vi "VibratomeGUI.vi"() -> ()   [LabVIEW 2014]
uses:
  Hardware/Table Stage/Controls/Translation Stage Cluster.ctl
  General/Controls/Translation Stage Types.ctl
  General/Controls/Translation Stage Quick Status.ctl
  General/Controls/Translation Stage Quick Controls.ctl
  General/Controls/Queue Manager Actions.ctl
  General/Controls/MessagePacket.ctl
  General/Controls/QueueNames.ctl
  <vilib>/Utility/miscctls.llb/LVPointTypeDef.ctl
  Hardware/Table Stage/Controls/Motion Translation Module Control.ctl
  General/Controls/Set Get Controls.ctl
panel:
  in  "Z STEP MOTION":enum16{"Fine", "Course", "Extra Course"}(ring)
  in  "Stop Button":bool
  in  "Slice":bool
  in  "Vibratome Controls":T1
  out "Message":string
  in  "Z Ctrl":T2
  out "Z Status":T3
  in  "Y Ctrl":T2
  out "Y Status":T3
  in  "X Ctrl":T2
  out "X Status":T3
  in  "XY STEP MOTION":enum16{"Fine", "Course", "Extra Course"}(ring)
  out "Cluster":cluster{"X":T4, "Y":T4, "Z":T4}
  in  "Exit":bool
  out "Processor Error Out":errorcluster
  out "GUI Error Out":errorcluster
  # "Vibratome Controls"
  # "Z Axis"
  # "Y Axis"
  # "X Axis"
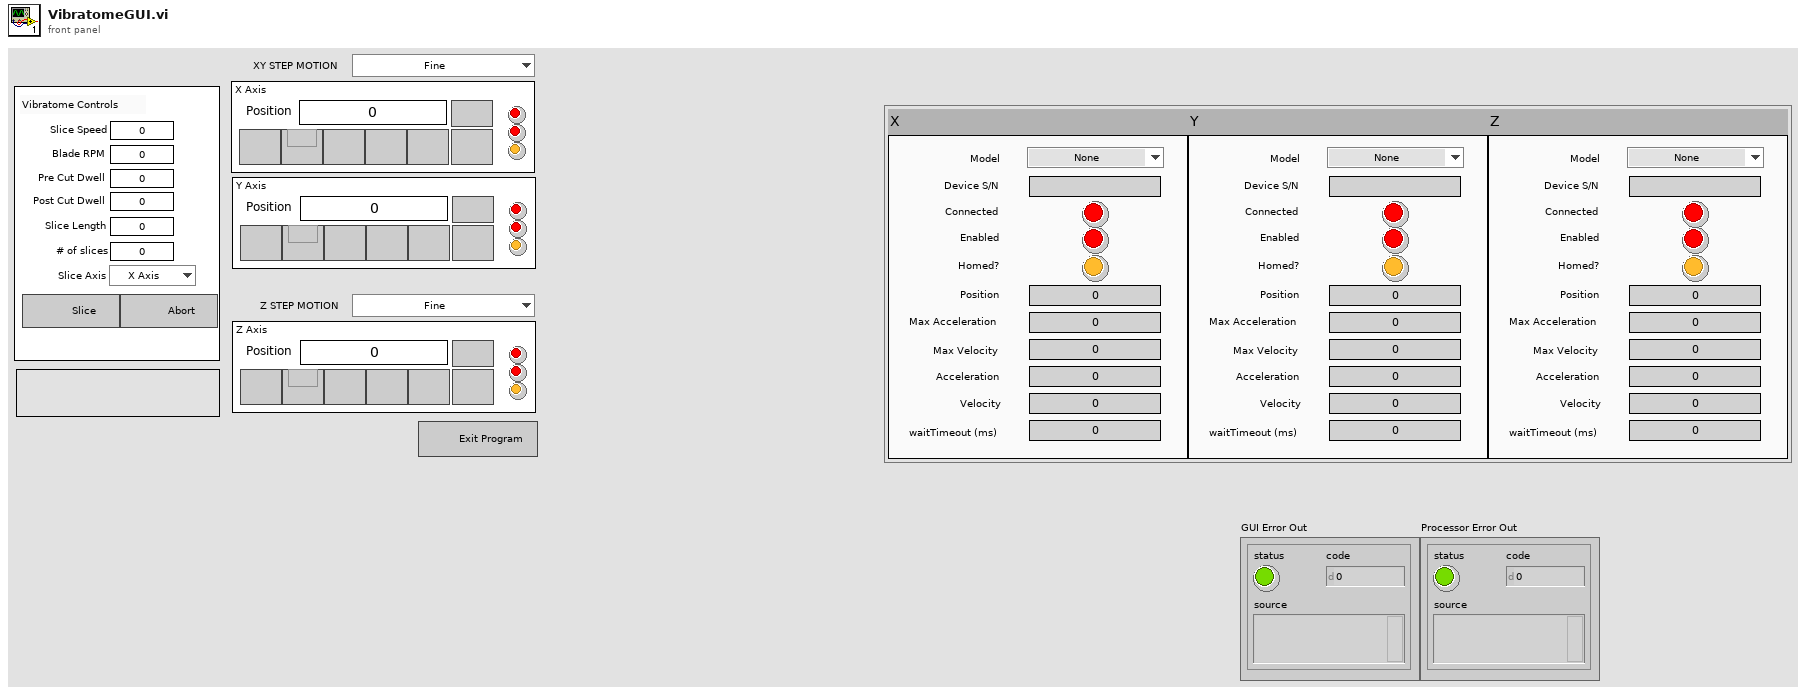
[diagram p1: front panel]
types:
  T1 = cluster{"Pre Cut Dwell":dbl, "Blade RPM":u16, "Slice Speed":dbl, "Post Cut Dwell":dbl, "Slice Length":dbl, "# of slices":dbl, "Slice Axis":enum16{"X Axis", "Y Axis", "Z Axis"}}
  T2 = typedef "Translation Stage Quick Controls.ctl" = cluster{"Position":dbl, "Next Button":bool, "Last Button":bool, "Previous Button":bool, "First Button":bool, "Home Button":bool, "Go":bool, "Settings Button":bool}
  T3 = typedef "Translation Stage Quick Status.ctl" = cluster{"Is.Enabled?":bool, "Is.Connected?":bool, "Is.Homed?":bool}
  T4 = typedef "Translation Stage Cluster.ctl" = cluster{"Position":dbl, "Is.Enabled?":bool, "Is.Connected?":bool, "Device SN":string, "AccelerationMaximum":dbl, "VelocityMaximum":dbl, "Acceleration":dbl, "Velocity":dbl, "waitTimeout (ms)":i32, "Model":T5, "Is.Homed?":bool}
  T5 = typedef "Translation Stage Types.ctl" = enum16{"None", "Thorlabs LTS", "Thorlabs MLJ"}
  T6 = typedef "MessagePacket.ctl" = cluster{"Message":string, "Parameter":variant}
  T7 = typedef "Queue Manager Actions.ctl" = enum16{"Init", "Enqueue", "Enqueue All", "Preview Queue", "Dequeue", "Get Status", "Flush Queue", "Flush All Queues", "Release All Queues", "Release Queue", "Enqueue at Opposite End"}
  T8 = typedef "QueueNames.ctl" = enum16{"Main GUI", "Main Scan Processor", "Main Display", "Main Table Stage GUI", "Main Table Stage Proc.", "Scan Engine", "Vibratome GUI", "Vibratome Processor", "Slice Engine"}
  T9 = typedef "LVPointTypeDef.ctl" = cluster{"Horizontal":i16, "Vertical":i16}
  T10 = enum16{"Set Configuration", "Get Configuration", "Enable Motor", "Disable Motor", "Get Status", "Open Session", "Close Session", "Set Limits", "Get Limits"}
  T11 = typedef "Set Get Controls.ctl" = enum16{"Set", "Get"}
  T12 = typedef "Motion Translation Module Control.ctl" = enum16{"Init", "Home", "Status", "Velocity/Accel", "Position", "Jog", "Stop", "Uninit", "Enable", "Disable"}
  T13 = cluster{"X Stage":T4, "Y Stage":T4, "Z Stage":T4}
  T14 = typedef "System Parameters.ctl" = cluster{"OCT":cluster{"Focal Length":dbl[unit]}, "Vibratome":cluster{"Z Bottom [mm]":dbl, "Pre Cut Dwell [s]":dbl, "Blade Frequency [RPM]":u16, "Slice Speed [mm/s]":dbl, "Post Cut Dwell [s]":dbl, "Ramp Time [s]":dbl, "Start X [mm]":dbl, "Start Y [mm]":dbl, "Slice Length [mm]":dbl, "Slice Axis":enum16{"X Axis", "Y Axis", "Z Axis"}, "Controller VISA Ref":refnum<visa-resource-name>}, "Table Stages":cluster{"X Stage":T4, "Y Stage":T4, "Z Stage":T4}}
  T15 = cluster{"Z Bottom [mm]":dbl, "Pre Cut Dwell [s]":dbl, "Blade Frequency [RPM]":u16, "Slice Speed [mm/s]":dbl, "Post Cut Dwell [s]":dbl, "Ramp Time [s]":dbl, "Start X [mm]":dbl, "Start Y [mm]":dbl, "Slice Length [mm]":dbl, "Slice Axis":enum16{"X Axis", "Y Axis", "Z Axis"}, "Controller VISA Ref":refnum<visa-resource-name>}
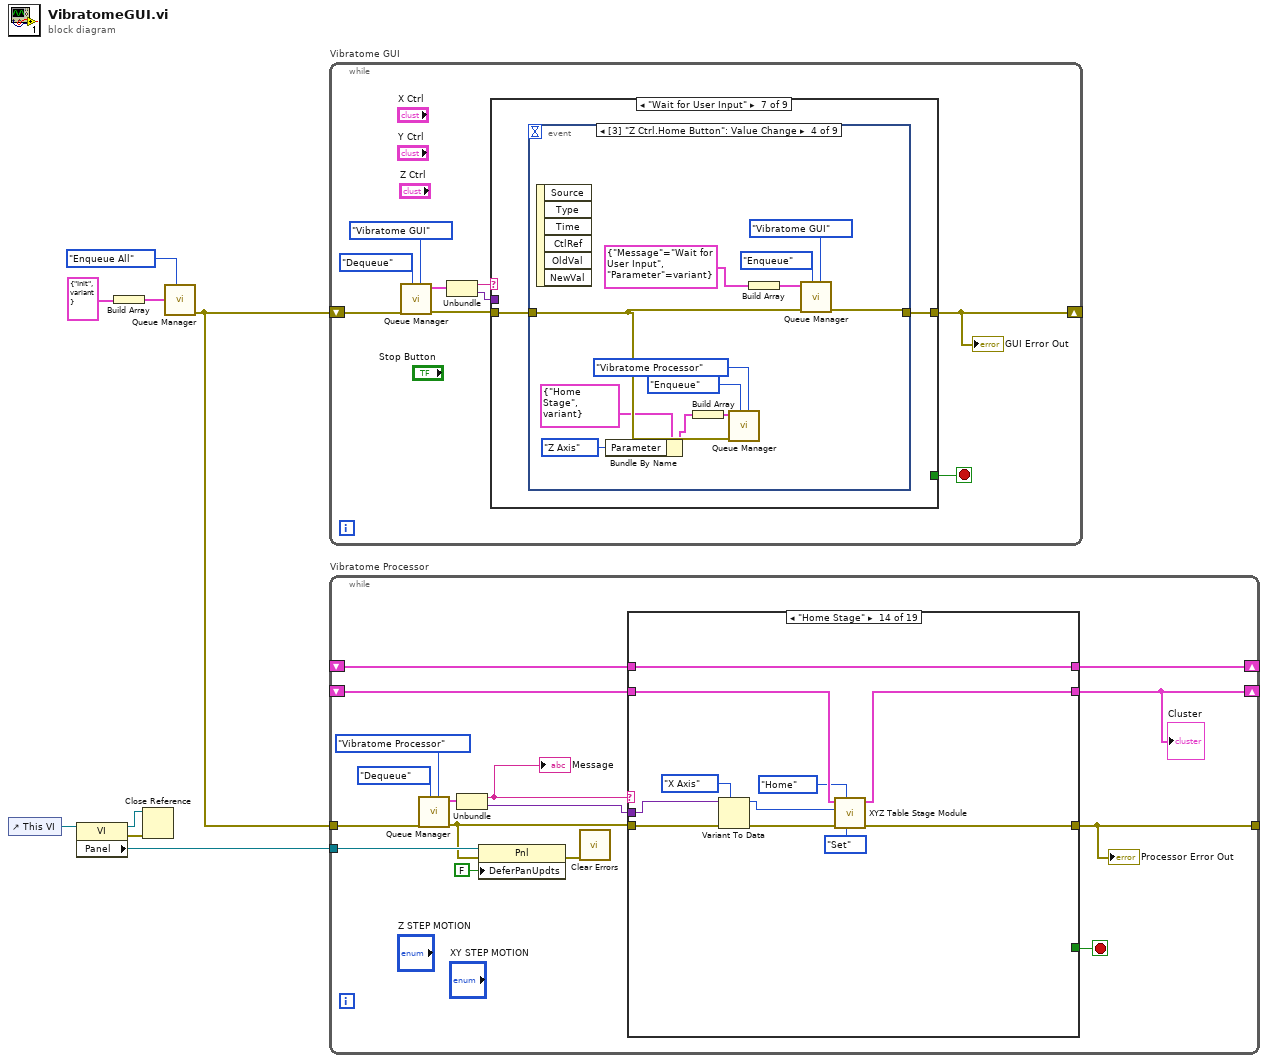
[diagram p0: block diagram]
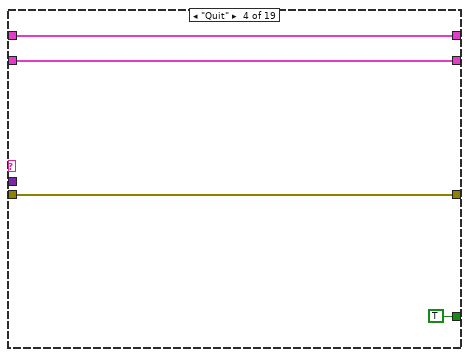
[diagram p5: hidden frame]
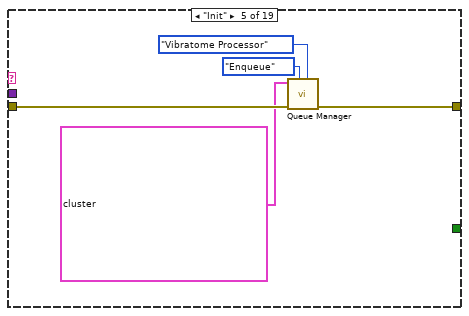
[diagram p6: hidden frame]
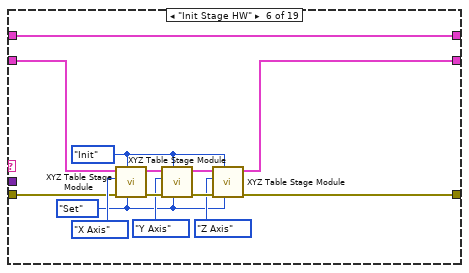
[diagram p7: hidden frame]
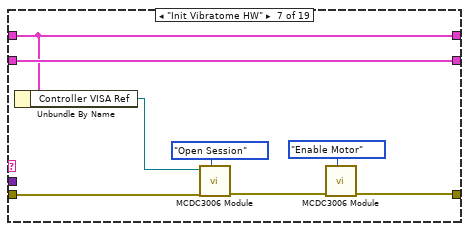
[diagram p8: hidden frame]
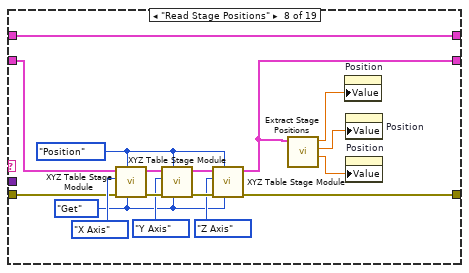
[diagram p9: hidden frame]
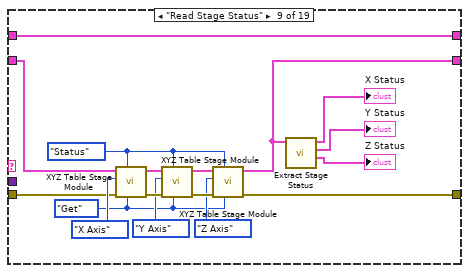
[diagram p10: hidden frame]
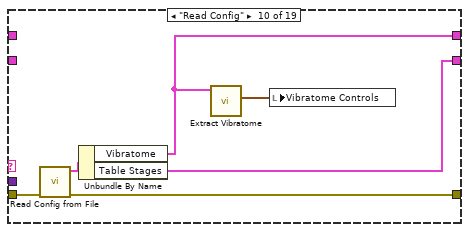
[diagram p11: hidden frame]
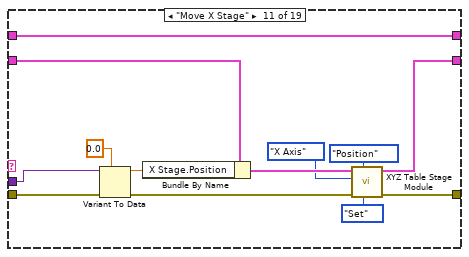
[diagram p12: hidden frame]
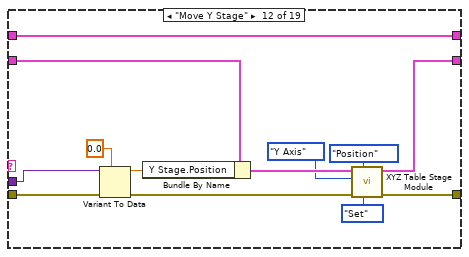
[diagram p13: hidden frame]
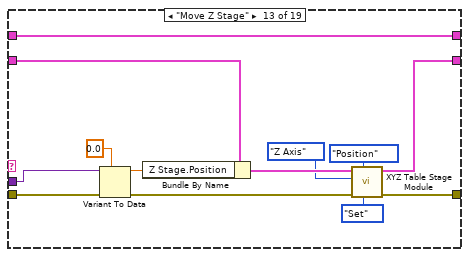
[diagram p14: hidden frame]
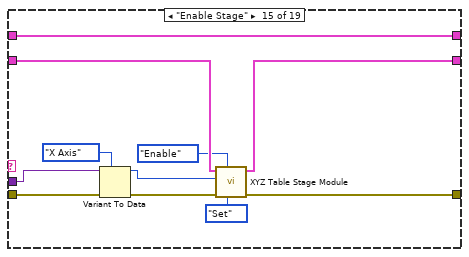
[diagram p15: hidden frame]
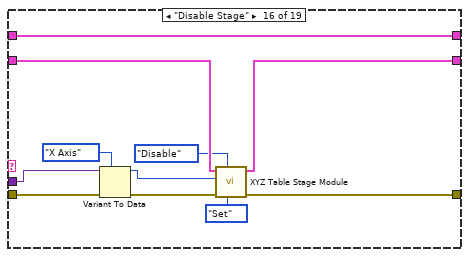
[diagram p16: hidden frame]
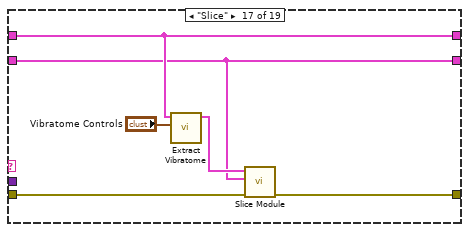
[diagram p17: hidden frame]
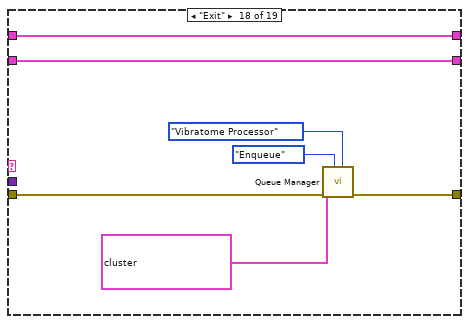
[diagram p18: hidden frame]
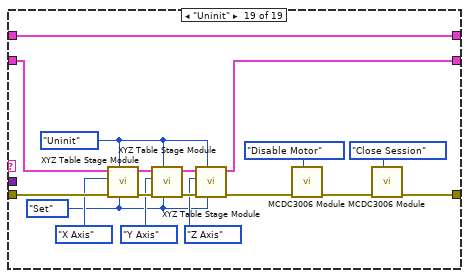
[diagram p19: hidden frame]
diagram:
  n1 = control-ref of="This VI"() -> (w4:refnum<vi>)
  n2 = property class="VI"(reference=w4) -> (reference out=w2:refnum<vi>, error out=w3:errorcluster, "Panel"=w1:refnum<vi>)  [unwired: 1 in]
  n3 = Build Array(T6 {"Message"="Init", "Parameter"=variant} ("Message Packet [In]")) -> (w6:T6[])
  n4 = Close Reference(reference=w2, error in (no error)=w3) -> ()  [unwired: 1 out]
  n5 = call "Queue Manager.vi"("Action"=Queue_Manager_Actions."Enqueue All", "Message Packet Array"=w6) -> ("Error Out"=w5:errorcluster)  [unwired: 7 in, 2 out]
  n6 = while "Vibratome GUI" {
    shift-right: [w17] -> _
    shift-left: w5 -> [w15]
    stop <- w10 stop-if-true
    n7 = call "Queue Manager.vi"("Queue Name"=QueueNames."Vibratome GUI", "Action"=Queue_Manager_Actions."Dequeue", "Error In"=w15) -> ("Error Out"=w14:errorcluster, "Message Packet [Out]"=w13:T6)  [unwired: 6 in, 1 out]
    n8 = Unbundle(w13) -> ("Message"=w12:string, "Parameter"=w11:variant)
    n9 = case shown="\"Wait for User Input\"" w12 {
      tunnel: w14 -> [w18 w19 w24 w25 w26 w27 w29 w126 w139]
      tunnel: [w18 w20 w24 w25 w26 w27 w28 w127 w139] -> w17
      tunnel: w11 -> [_ _ _ _ _ _ _ _ _]
      tunnel: [_ _ _ _ _ _ _ _ TRUE] -> w10
      frame "Unknown", Default {
      }
      frame "Init" {
        n10 = call "Queue Manager.vi"("Queue Name"=QueueNames."Vibratome GUI", "Action"=Queue_Manager_Actions."Enqueue", "Error In"=w19, "Message Packet Array"=T6[] [{"Message"="Init Variables", "Parameter"=variant}, {"Message"="Set Front Panel", "Parameter"=variant}, {"Message"="Load User Settings", "Parameter"=variant}, {"Message"="Configure Hardware", "Parameter"=variant}, {"Message"="Wait for Complete", "Parameter"=variant}, {"Message"="Wait for User Input", "Parameter"=variant}]) -> ("Error Out"=w20:errorcluster)  [unwired: 5 in, 2 out]
      }
      frame "Init Variables" {
      }
      frame "Load User Settings" {
      }
      frame "Configure Hardware" {
      }
      frame "Wait for Complete" {
      }
      frame "Wait for User Input" {
        n11 = event shown="[3] \"Z Ctrl.Home Button\": Value Change" {
          selector: _ -> [_ _ _ _ _ _ _ _ _]
          dyn-events: _ -> [_ _ _ _ _ _ _ _ _]
          timeout: _ -> [_ _ _ _ _ _ _ _ _]
          tunnel: w29 -> [w30 w38 w50 w62 w70 w73 w95 w110 w125]
          tunnel: [w30 w37 w49 w61 w69 w78 w82 w97 w112] -> w28
          event Timeout {
            n12 = event-data() -> ()  [unwired: 1 in, 3 out]
          }
          event Value Change {
            n13 = event-data() -> ()  [unwired: 1 in, 6 out]
            n14 = Bundle By Name(cluster=T6 {"Message"="Home Stage", "Parameter"=variant} ("Message Packet [In]"), "Parameter"=enum16{"X Axis", "Y Axis", "Z Axis"}."X Axis" ("Axis")) -> (w32:T6)
            n15 = Build Array(w32) -> (w33:T6[])
            n16 = call "Queue Manager.vi"("Queue Name"=QueueNames."Vibratome Processor", "Action"=Queue_Manager_Actions."Enqueue", "Error In"=w38, "Message Packet Array"=w33) -> ()  [unwired: 5 in, 3 out]
            n17 = Build Array(T6 {"Message"="Wait for User Input", "Parameter"=variant} ("Message Packet [In]")) -> (w35:T6[])
            n18 = call "Queue Manager.vi"("Queue Name"=QueueNames."Vibratome GUI", "Action"=Queue_Manager_Actions."Enqueue", "Error In"=w38, "Message Packet Array"=w35) -> ("Error Out"=w37:errorcluster)  [unwired: 5 in, 2 out]
          }
          event Value Change {
            n19 = event-data() -> ()  [unwired: 1 in, 6 out]
            n20 = Bundle By Name(cluster=T6 {"Message"="Home Stage", "Parameter"=variant} ("Message Packet [In]"), "Parameter"=enum16{"X Axis", "Y Axis", "Z Axis"}."Y Axis" ("Axis")) -> (w44:T6)
            n21 = Build Array(w44) -> (w45:T6[])
            n22 = call "Queue Manager.vi"("Queue Name"=QueueNames."Vibratome Processor", "Action"=Queue_Manager_Actions."Enqueue", "Error In"=w50, "Message Packet Array"=w45) -> ()  [unwired: 5 in, 3 out]
            n23 = Build Array(T6 {"Message"="Wait for User Input", "Parameter"=variant} ("Message Packet [In]")) -> (w47:T6[])
            n24 = call "Queue Manager.vi"("Queue Name"=QueueNames."Vibratome GUI", "Action"=Queue_Manager_Actions."Enqueue", "Error In"=w50, "Message Packet Array"=w47) -> ("Error Out"=w49:errorcluster)  [unwired: 5 in, 2 out]
          }
          event Value Change {
            n25 = event-data() -> ()  [unwired: 1 in, 6 out]
            n26 = Bundle By Name(cluster=T6 {"Message"="Home Stage", "Parameter"=variant} ("Message Packet [In]"), "Parameter"=enum16{"X Axis", "Y Axis", "Z Axis"}."Z Axis" ("Axis")) -> (w56:T6)
            n27 = Build Array(w56) -> (w57:T6[])
            n28 = call "Queue Manager.vi"("Queue Name"=QueueNames."Vibratome Processor", "Action"=Queue_Manager_Actions."Enqueue", "Error In"=w62, "Message Packet Array"=w57) -> ()  [unwired: 5 in, 3 out]
            n29 = Build Array(T6 {"Message"="Wait for User Input", "Parameter"=variant} ("Message Packet [In]")) -> (w59:T6[])
            n30 = call "Queue Manager.vi"("Queue Name"=QueueNames."Vibratome GUI", "Action"=Queue_Manager_Actions."Enqueue", "Error In"=w62, "Message Packet Array"=w59) -> ("Error Out"=w61:errorcluster)  [unwired: 5 in, 2 out]
          }
          event Panel Close; Application Instance Close; "Exit": Value Change {
            n31 = event-data() -> ()  [unwired: 1 in, 3 out]
            n32 = Build Array(T6 {"Message"="Exit", "Parameter"=variant} ("Message Packet [In]")) -> (w67:T6[])
            n33 = call "Queue Manager.vi"("Action"=Queue_Manager_Actions."Enqueue All", "Error In"=w70, "Message Packet Array"=w67) -> ("Error Out"=w69:errorcluster)  [unwired: 6 in, 2 out]
          }
          event "Slice": Value Change {
            n34 = event-data() -> ()  [unwired: 1 in, 6 out]
            n35 = Build Array(T6 {"Message"="Wait for User Input", "Parameter"=variant} ("Message Packet [In]")) -> (w76:T6[])
            n36 = call "Queue Manager.vi"("Queue Name"=QueueNames."Vibratome GUI", "Action"=Queue_Manager_Actions."Enqueue", "Error In"=w73, "Message Packet Array"=w76) -> ("Error Out"=w78:errorcluster)  [unwired: 5 in, 2 out]
            n37 = call "Queue Manager.vi"("Queue Name"=QueueNames."Vibratome Processor", "Action"=Queue_Manager_Actions."Enqueue", "Error In"=w73, "Message Packet Array"=T6[] [{"Message"="Slice", "Parameter"=variant}, {"Message"="Finished", "Parameter"=variant}]) -> ()  [unwired: 5 in, 3 out]
          }
          event Value Change {
            n38 = event-data() -> ()  [unwired: 1 in, 1 out]
            n39 = property on="Position" class="DigNum (strict)"(error in=w95) -> (error out=w92:errorcluster, "Value"=w90:dbl)  [unwired: 1 in, 1 out]
            n40 = Bundle By Name(cluster=T6 {"Message"="Move X Stage", "Parameter"=variant} ("Message Packet [In]"), "Parameter"=w90) -> (w89:T6)
            n41 = Build Array(w89, T6 {"Message"="Finished", "Parameter"=variant} ("Message Packet [In]")) -> (w88:T6[])
            n42 = call "Queue Manager.vi"("Queue Name"=QueueNames."Vibratome Processor", "Action"=Queue_Manager_Actions."Enqueue", "Error In"=w92, "Message Packet Array"=w88) -> ("Error Out"=w83:errorcluster)  [unwired: 5 in, 2 out]
            n43 = Build Array(T6 {"Message"="Wait for User Input", "Parameter"=variant} ("Message Packet [In]")) -> (w84:T6[])
            n44 = call "Queue Manager.vi"("Queue Name"=QueueNames."Vibratome GUI", "Action"=Queue_Manager_Actions."Enqueue", "Error In"=w83, "Message Packet Array"=w84) -> ("Error Out"=w82:errorcluster)  [unwired: 5 in, 2 out]
          }
          event Value Change {
            n45 = event-data() -> ()  [unwired: 1 in, 1 out]
            n46 = property on="Position" class="DigNum (strict)"(error in=w110) -> (error out=w107:errorcluster, "Value"=w105:dbl)  [unwired: 1 in, 1 out]
            n47 = Bundle By Name(cluster=T6 {"Message"="Move Y Stage", "Parameter"=variant} ("Message Packet [In]"), "Parameter"=w105) -> (w104:T6)
            n48 = Build Array(w104, T6 {"Message"="Finished", "Parameter"=variant} ("Message Packet [In]")) -> (w103:T6[])
            n49 = call "Queue Manager.vi"("Queue Name"=QueueNames."Vibratome Processor", "Action"=Queue_Manager_Actions."Enqueue", "Error In"=w107, "Message Packet Array"=w103) -> ("Error Out"=w98:errorcluster)  [unwired: 5 in, 2 out]
            n50 = Build Array(T6 {"Message"="Wait for User Input", "Parameter"=variant} ("Message Packet [In]")) -> (w99:T6[])
            n51 = call "Queue Manager.vi"("Queue Name"=QueueNames."Vibratome GUI", "Action"=Queue_Manager_Actions."Enqueue", "Error In"=w98, "Message Packet Array"=w99) -> ("Error Out"=w97:errorcluster)  [unwired: 5 in, 2 out]
          }
          event Value Change {
            n52 = event-data() -> ()  [unwired: 1 in, 1 out]
            n53 = property on="Position" class="DigNum (strict)"(error in=w125) -> (error out=w122:errorcluster, "Value"=w120:dbl)  [unwired: 1 in, 1 out]
            n54 = Bundle By Name(cluster=T6 {"Message"="Move Z Stage", "Parameter"=variant} ("Message Packet [In]"), "Parameter"=w120) -> (w119:T6)
            n55 = Build Array(w119, T6 {"Message"="Finished", "Parameter"=variant} ("Message Packet [In]")) -> (w118:T6[])
            n56 = call "Queue Manager.vi"("Queue Name"=QueueNames."Vibratome Processor", "Action"=Queue_Manager_Actions."Enqueue", "Error In"=w122, "Message Packet Array"=w118) -> ("Error Out"=w113:errorcluster)  [unwired: 5 in, 2 out]
            n57 = Build Array(T6 {"Message"="Wait for User Input", "Parameter"=variant} ("Message Packet [In]")) -> (w114:T6[])
            n58 = call "Queue Manager.vi"("Queue Name"=QueueNames."Vibratome GUI", "Action"=Queue_Manager_Actions."Enqueue", "Error In"=w113, "Message Packet Array"=w114) -> ("Error Out"=w112:errorcluster)  [unwired: 5 in, 2 out]
          }
        }
      }
      frame "Set Front Panel" {
        n59 = control-ref of="This VI"() -> (w128:refnum<vi>)
        n60 = property class="VI"(reference=w128, error in=w126) -> (error out=w130:errorcluster, "Panel"=w133:refnum<vi>)  [unwired: 1 out]
        n61 = property class="Pnl"(reference=w133, error in=w130) -> (error out=w131:errorcluster, "Panes[]"=w132:refnum<vi>[])  [unwired: 1 out]
        n62 = for {
          tunnel: w132 -> [w137] mode=indexing
          tunnel: w131 -> [w135]
          tunnel: [w134] -> w129 mode=indexing
          n63 = property class="Pane"(reference=w137, error in=w135, "Origin"=T9 {"Horizontal"=0, "Vertical"=0}) -> (error out=w134:errorcluster)  [unwired: 1 out]
        }
        n64 = Merge Errors(w129) -> (w127:errorcluster)
      }
      frame "Exit" {
      }
    }
    "GUI Error Out" <- w17
  }
  n65 = while "Vibratome Processor" {
    tunnel: w5 -> [w153]
    tunnel: [w155] -> _
    shift-right: [w144] -> _
    shift-left: _ -> [w147]
    shift-right: [w146] -> _
    shift-left: _ -> [w145]
    tunnel: w1 -> [w143]
    stop <- w149 stop-if-true
    n66 = call "Queue Manager.vi"("Queue Name"=QueueNames."Vibratome Processor", "Action"=Queue_Manager_Actions."Dequeue", "Error In"=w153) -> ("Error Out"=w141:errorcluster, "Message Packet [Out]"=w152:T6)  [unwired: 6 in, 1 out]
    n67 = Unbundle(w152) -> ("Message"=w151:string, "Parameter"=w150:variant)
    "Message" <- w151
    n68 = property class="Pnl"(reference=w143, error in=w141, "DeferPanUpdts"=FALSE ("Defer Panel Updates")) -> (error out=w140:errorcluster)  [unwired: 1 out]
    n69 = call <vilib>:"Clear Errors.vi"("error in (no error)"=w140) -> ()  [unwired: 5 in, 2 out]
    n70 = case shown="\"Home Stage\"" w151 {
      tunnel: w141 -> [w158 w161 w162 w166 w173 w177 w193 w202 w219 w235 w248 w261 w274 w285 w296 w307 w312 w318 w338]
      tunnel: [w158 w161 w162 w166 w172 w185 w189 w210 w227 w232 w247 w260 w273 w284 w295 w306 w311 w317 w322] -> w155
      tunnel: w150 -> [_ _ _ _ _ _ _ _ _ _ w245 w258 w271 w282 w293 w304 _ _ _]
      tunnel: [_ _ _ TRUE _ _ _ _ _ _ _ _ _ _ _ _ _ _ _] -> w149
      tunnel: [w157 w160 w164 w168 _ w174 w195 w196 w217 w233 w244 w257 w270 w278 w289 w300 w309 w319 w331] -> w144
      tunnel: w147 -> [w157 w160 w164 w168 _ w176 w195 w201 w218 _ w240 w253 w266 w279 w290 w301 w309 w319 w334]
      tunnel: [w156 w159 w163 w167 _ w175 w191 w200 w213 w231 w236 w249 w262 w275 w286 w297 w313 w320 w325] -> w146
      tunnel: w145 -> [w156 w159 w163 w167 _ w175 w191 w200 w213 _ w236 w249 w262 w275 w286 w297 w313 w320 w325]
      frame "Unknown", Default {
      }
      frame "Finished Init" {
      }
      frame "Finished" {
      }
      frame "Quit" {
      }
      frame "Init" {
        n71 = call "Queue Manager.vi"("Queue Name"=QueueNames."Vibratome Processor", "Action"=Queue_Manager_Actions."Enqueue", "Error In"=w173, "Message Packet Array"=T6[] [{"Message"="Read Config", "Parameter"=variant}, {"Message"="Init Stage HW", "Parameter"=variant}, {"Message"="Read Stage Status", "Parameter"=variant}, {"Message"="Read Stage Positions", "Parameter"=variant}, {"Message"="Init Vibratome HW", "Parameter"=variant}, {"Message"="Finished Init", "Parameter"=variant}]) -> ("Error Out"=w172:errorcluster)  [unwired: 5 in, 2 out]
      }
      frame "Init Stage HW" {
        w178 = Set_Get_Controls."Set" ("Set/Get")
        w184 = Motion_Translation_Module_Control."Init" ("Action")
        n72 = call "XYZ Table Stage Module.vi"("Set/Get"=w178, "Action"=w184, "Error In"=w177, "Axis"=enum16{"X Axis", "Y Axis", "Z Axis"}."X Axis", "Table Stages"=w176) -> ("Error Out"=w187:errorcluster, "Table Stages Out"=w183:T13)  [unwired: 5 in]
        n73 = call "XYZ Table Stage Module.vi"("Set/Get"=w178, "Action"=w184, "Error In"=w187, "Axis"=enum16{"X Axis", "Y Axis", "Z Axis"}."Y Axis", "Table Stages"=w183) -> ("Error Out"=w186:errorcluster, "Table Stages Out"=w182:T13)  [unwired: 5 in]
        n74 = call "XYZ Table Stage Module.vi"("Set/Get"=w178, "Action"=w184, "Error In"=w186, "Axis"=enum16{"X Axis", "Y Axis", "Z Axis"}."Z Axis", "Table Stages"=w182) -> ("Error Out"=w185:errorcluster, "Table Stages Out"=w174:T13)  [unwired: 5 in]
      }
      frame "Init Vibratome HW" {
        n75 = Unbundle By Name(w191) -> ("Controller VISA Ref"=w190:refnum<visa-resource-name>)
        n76 = call "MCDC3006 Module.vi"("Actions"=T10."Open Session", "Error In"=w193, "VISA resource name"=w190) -> ("Error Out"=w192:errorcluster)  [unwired: 4 in, 4 out]
        n77 = call "MCDC3006 Module.vi"("Actions"=T10."Enable Motor", "Error In"=w192) -> ("Error Out"=w189:errorcluster)  [unwired: 5 in, 4 out]
      }
      frame "Read Stage Positions" {
        w203 = Set_Get_Controls."Get" ("Set/Get")
        w209 = Motion_Translation_Module_Control."Position" ("Action")
        n78 = call "XYZ Table Stage Module.vi"("Set/Get"=w203, "Action"=w209, "Error In"=w202, "Axis"=enum16{"X Axis", "Y Axis", "Z Axis"}."X Axis", "Table Stages"=w201) -> ("Error Out"=w212:errorcluster, "Table Stages Out"=w208:T13)  [unwired: 5 in]
        n79 = call "XYZ Table Stage Module.vi"("Set/Get"=w203, "Action"=w209, "Error In"=w212, "Axis"=enum16{"X Axis", "Y Axis", "Z Axis"}."Y Axis", "Table Stages"=w208) -> ("Error Out"=w211:errorcluster, "Table Stages Out"=w207:T13)  [unwired: 5 in]
        n80 = call "XYZ Table Stage Module.vi"("Set/Get"=w203, "Action"=w209, "Error In"=w211, "Axis"=enum16{"X Axis", "Y Axis", "Z Axis"}."Z Axis", "Table Stages"=w207) -> ("Error Out"=w210:errorcluster, "Table Stages Out"=w196:T13)  [unwired: 5 in]
        n81 = call "Extract Stage Positions.vi"("Table Stages"=w196) -> ("Z Stage.Position"=w197:dbl, "Y Stage.Position"=w198:dbl, "X Stage.Position"=w199:dbl)  [unwired: 8 in]
        n82 = property on="Position" class="DigNum (strict)"("Value"=w199) -> ()  [unwired: 2 in, 2 out]
        n83 = property on="Position" class="DigNum (strict)"("Value"=w198) -> ()  [unwired: 2 in, 2 out]
        n84 = property on="Position" class="DigNum (strict)"("Value"=w197) -> ()  [unwired: 2 in, 2 out]
      }
      frame "Read Stage Status" {
        w220 = Set_Get_Controls."Get" ("Set/Get")
        w226 = Motion_Translation_Module_Control."Status" ("Action")
        n85 = call "XYZ Table Stage Module.vi"("Set/Get"=w220, "Action"=w226, "Error In"=w219, "Axis"=enum16{"X Axis", "Y Axis", "Z Axis"}."X Axis", "Table Stages"=w218) -> ("Error Out"=w229:errorcluster, "Table Stages Out"=w225:T13)  [unwired: 5 in]
        n86 = call "XYZ Table Stage Module.vi"("Set/Get"=w220, "Action"=w226, "Error In"=w229, "Axis"=enum16{"X Axis", "Y Axis", "Z Axis"}."Y Axis", "Table Stages"=w225) -> ("Error Out"=w228:errorcluster, "Table Stages Out"=w224:T13)  [unwired: 5 in]
        n87 = call "XYZ Table Stage Module.vi"("Set/Get"=w220, "Action"=w226, "Error In"=w228, "Axis"=enum16{"X Axis", "Y Axis", "Z Axis"}."Z Axis", "Table Stages"=w224) -> ("Error Out"=w227:errorcluster, "Table Stages Out"=w217:T13)  [unwired: 5 in]
        n88 = call "Extract Stage Status.vi"("Table Stages"=w217) -> ("Z Stage"=→"Z Status":T3, "Y Stage"=→"Y Status":T3, "X Stage"=→"X Status":T3)  [unwired: 8 in]
      }
      frame "Read Config" {
        n89 = call "Read Config from File.vi"("error in (no error)"=w235) -> ("error out"=w232:errorcluster, "System Parameters"=w234:T14)  [unwired: 9 in]
        n90 = Unbundle By Name(w234) -> ("Vibratome"=w231:T15, "Table Stages"=w233:T13)
        n91 = call "Extract Vibratome.vi"("Vibratome"=w231) -> ("Vibratome Controls Out"=w230:T1)  [unwired: 9 in, 1 out]
        n92 = local write "Vibratome Controls"(w230) -> ()
      }
      frame "Move X Stage" {
        n93 = Variant To Data(error in=w248, type=0.0 ("Value"), Variant=w245) -> (data=w239:dbl, error out=w246:errorcluster)
        n94 = Bundle By Name(cluster=w240, "X Stage.Position"=w239) -> (w238:T13)
        n95 = call "XYZ Table Stage Module.vi"("Set/Get"=Set_Get_Controls."Set", "Action"=Motion_Translation_Module_Control."Position", "Error In"=w246, "Axis"=enum16{"X Axis", "Y Axis", "Z Axis"}."X Axis", "Table Stages"=w238) -> ("Error Out"=w247:errorcluster, "Table Stages Out"=w244:T13)  [unwired: 5 in]
      }
      frame "Move Y Stage" {
        n96 = Variant To Data(error in=w261, type=0.0 ("Value"), Variant=w258) -> (data=w252:dbl, error out=w259:errorcluster)
        n97 = Bundle By Name(cluster=w253, "Y Stage.Position"=w252) -> (w251:T13)
        n98 = call "XYZ Table Stage Module.vi"("Set/Get"=Set_Get_Controls."Set", "Action"=Motion_Translation_Module_Control."Position", "Error In"=w259, "Axis"=enum16{"X Axis", "Y Axis", "Z Axis"}."Y Axis", "Table Stages"=w251) -> ("Error Out"=w260:errorcluster, "Table Stages Out"=w257:T13)  [unwired: 5 in]
      }
      frame "Move Z Stage" {
        n99 = Variant To Data(error in=w274, type=0.0 ("Value"), Variant=w271) -> (data=w265:dbl, error out=w272:errorcluster)
        n100 = Bundle By Name(cluster=w266, "Z Stage.Position"=w265) -> (w264:T13)
        n101 = call "XYZ Table Stage Module.vi"("Set/Get"=Set_Get_Controls."Set", "Action"=Motion_Translation_Module_Control."Position", "Error In"=w272, "Axis"=enum16{"X Axis", "Y Axis", "Z Axis"}."Z Axis", "Table Stages"=w264) -> ("Error Out"=w273:errorcluster, "Table Stages Out"=w270:T13)  [unwired: 5 in]
      }
      frame "Home Stage" {
        n102 = Variant To Data(error in=w285, type=enum16{"X Axis", "Y Axis", "Z Axis"}."X Axis" ("Axis"), Variant=w282) -> (data=w280:enum16{"X Axis", "Y Axis", "Z Axis"}, error out=w283:errorcluster)
        n103 = call "XYZ Table Stage Module.vi"("Set/Get"=Set_Get_Controls."Set", "Action"=Motion_Translation_Module_Control."Home", "Error In"=w283, "Axis"=w280, "Table Stages"=w279) -> ("Error Out"=w284:errorcluster, "Table Stages Out"=w278:T13)  [unwired: 5 in]
      }
      frame "Enable Stage" {
        n104 = Variant To Data(error in=w296, type=enum16{"X Axis", "Y Axis", "Z Axis"}."X Axis" ("Axis"), Variant=w293) -> (data=w291:enum16{"X Axis", "Y Axis", "Z Axis"}, error out=w294:errorcluster)
        n105 = call "XYZ Table Stage Module.vi"("Set/Get"=Set_Get_Controls."Set", "Action"=Motion_Translation_Module_Control."Enable", "Error In"=w294, "Axis"=w291, "Table Stages"=w290) -> ("Error Out"=w295:errorcluster, "Table Stages Out"=w289:T13)  [unwired: 5 in]
      }
      frame "Disable Stage" {
        n106 = Variant To Data(error in=w307, type=enum16{"X Axis", "Y Axis", "Z Axis"}."X Axis" ("Axis"), Variant=w304) -> (data=w302:enum16{"X Axis", "Y Axis", "Z Axis"}, error out=w305:errorcluster)
        n107 = call "XYZ Table Stage Module.vi"("Set/Get"=Set_Get_Controls."Set", "Action"=Motion_Translation_Module_Control."Disable", "Error In"=w305, "Axis"=w302, "Table Stages"=w301) -> ("Error Out"=w306:errorcluster, "Table Stages Out"=w300:T13)  [unwired: 5 in]
      }
      frame "Slice" {
        n108 = call "Extract Vibratome.vi"("Vibratome Controls In"="Vibratome Controls", "Vibratome"=w313) -> ("Vibratome Out"=w310:T15)  [unwired: 8 in, 1 out]
        n109 = call "Slice Module.vi"("Error In"=w312, "Table Stages"=w309, "Vibratome"=w310) -> ("Error Out"=w311:errorcluster)  [unwired: 6 in, 2 out]
      }
      frame "Exit" {
        n110 = call "Queue Manager.vi"("Queue Name"=QueueNames."Vibratome Processor", "Action"=Queue_Manager_Actions."Enqueue", "Error In"=w318, "Message Packet Array"=T6[] [{"Message"="Uninit", "Parameter"=variant}, {"Message"="Quit", "Parameter"=variant}]) -> ("Error Out"=w317:errorcluster)  [unwired: 5 in, 2 out]
      }
      frame "Uninit" {
        w326 = Set_Get_Controls."Set" ("Set/Get")
        w330 = Motion_Translation_Module_Control."Uninit" ("Action")
        n111 = call "XYZ Table Stage Module.vi"("Set/Get"=w326, "Action"=w330, "Error In"=w338, "Axis"=enum16{"X Axis", "Y Axis", "Z Axis"}."X Axis", "Table Stages"=w334) -> ("Error Out"=w336:errorcluster, "Table Stages Out"=w333:T13)  [unwired: 5 in]
        n112 = call "XYZ Table Stage Module.vi"("Set/Get"=w326, "Action"=w330, "Error In"=w336, "Axis"=enum16{"X Axis", "Y Axis", "Z Axis"}."Y Axis", "Table Stages"=w333) -> ("Error Out"=w337:errorcluster, "Table Stages Out"=w332:T13)  [unwired: 5 in]
        n113 = call "XYZ Table Stage Module.vi"("Set/Get"=w326, "Action"=w330, "Error In"=w337, "Axis"=enum16{"X Axis", "Y Axis", "Z Axis"}."Z Axis", "Table Stages"=w332) -> ("Error Out"=w335:errorcluster, "Table Stages Out"=w331:T13)  [unwired: 5 in]
        n114 = call "MCDC3006 Module.vi"("Actions"=T10."Disable Motor", "Error In"=w335) -> ("Error Out"=w324:errorcluster)  [unwired: 5 in, 4 out]
        n115 = call "MCDC3006 Module.vi"("Actions"=T10."Close Session", "Error In"=w324) -> ("Error Out"=w322:errorcluster)  [unwired: 5 in, 4 out]
      }
    }
    "Processor Error Out" <- w155
    "Cluster" <- w144
  }
